vi "ParseColorDisp.vi"(2 "text":string, 3 "text color(black)":u32(colorbox), 4 "Init?":bool) -> (1 "picture out":picture)   [LabVIEW 2015]
doc: "Parses a color display and returns a picture"
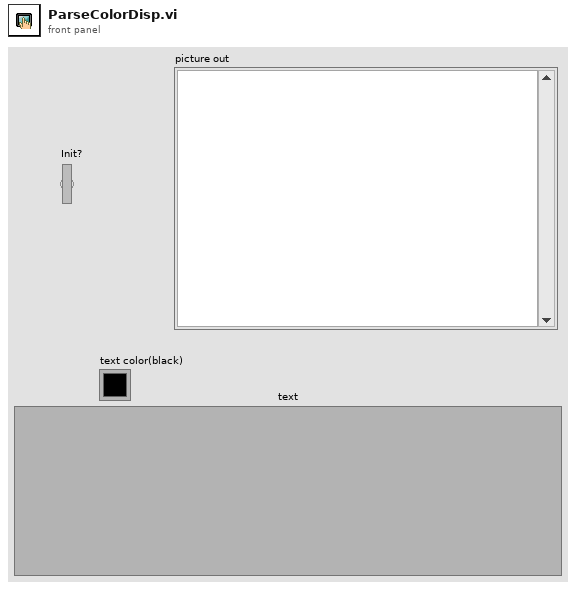
[diagram p1: front panel]
types:
  T1 = cluster{"left":i16, "top":i16, "right":i16, "bottom":i16}
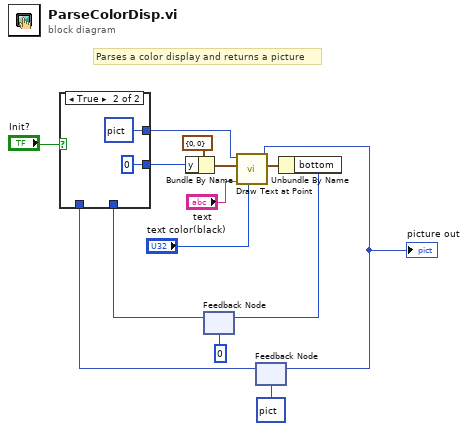
[diagram p0: block diagram]
diagram:
  # "Parses a color display and returns a picture"
  n1 = feedback #1(i16 0 ("bottom")) -> (w1:i16)
  n2 = feedback #2(picture data[5B] ("new picture")) -> (w3:picture)
  n3 = case shown="True" "Init?" {
    tunnel: w3 -> [w16 _]
    tunnel: [w16 picture data[5B] ("new picture")] -> w4
    tunnel: w1 -> [w15 _]
    tunnel: [w15 i16 0 ("bottom")] -> w2
    frame False {
    }
    frame True {
    }
  }
  n4 = Bundle By Name(cluster=cluster{"x":i16, "y":i16} {"x"=0, "y"=0} ("origin"), "y"=w2) -> (w14:cluster{"x":i16, "y":i16})
  n5 = call "Draw Text at Point.vi"("text color(black)"="text color(black)", "text"="text", "origin"=w14, "picture"=w4) -> ("text rect"=w12:T1, "new picture"=w6:picture)  [unwired: 6 in]
  "picture out" <- w6
  n6 = feedback-in #2(w6) -> ()
  n7 = Unbundle By Name(w12) -> ("bottom"=w9:i16)
  n8 = feedback-in #1(w9) -> ()
